vi "Offline Noise Reduction with Time Varying Filter.vi"() -> ()   [LabVIEW 2023]
doc: "This example shows the application of linear Time Frequency Analysis VIs in offline noise reduction applications. \n\nFor nonstationary signals whose spectral contents evolve over time, you usually use time-varying filters to reduce noise in the signals. The specification of a time-varying filter changes over time and is adaptable to signals. The Time Varying Filter (Thresholding) Express VI implements filtering with the following three steps: converting a signal into the time-frequency representation using the Gabor transform, removing noise in the time-frequency domain, and reconstructing the signal with noise reduced using the Gabor expansion. The Gabor transform-based filtering can be applied to both online and offline applications. \n\nThis example uses the Time Varying Filter (Thresholding) Express VI to reduce noise in a simulated chirp signal. \n\n<b>Instructions:</b>\n1) Run this VI.\n2) Compare the original <b>Noisy Signal</b> and <b>Denoised Signal</b>.\n3) Browse the Block Diagram of this example and double-click the Time Varying Filter (Thresholding) Express VI to observe the settings of the time-varying filter."
uses:
  <vilib>/addons/Time Frequency Analysis/typedefs.llb/TFA Data.ctl
  Instance           1 56Saved   Offline Noise Reduction with Time Varying Filter .vi
  <vilib>/addons/_Advanced Signal Processing/NI_AdvSigProcTFA.lvlib
panel:
  out "aspt-left-top":bool
  out "Signals":waveform(dbl)[](graph)
  # "Overview: Shows the application of linear Time Frequency Analysis VIs in offline noise reduction applications.\nRequirements: LabVIEW Full Development System, Advanced Signal Processing Toolkit\nInstructions: \n1. Run this VI.\n2. Compare the original Noisy Signal and Denoised Signal.\n3. Browse the block diagram of this example and double-click the Time Varying Filter (Thresholding) Express VI to observe the settings of the time-varying filter."
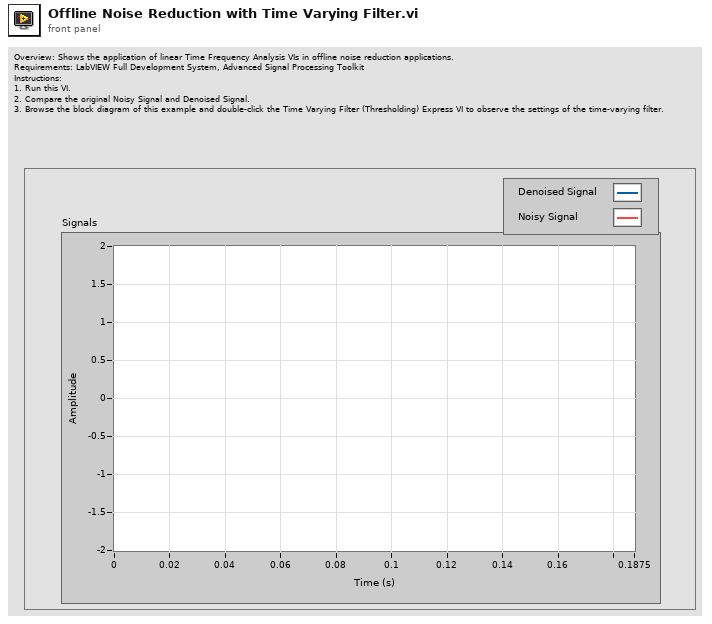
[diagram p1: front panel]
types:
  T1 = typedef "NI_AdvSigProcTFA.lvlib/TFA Data.ctl" = u16
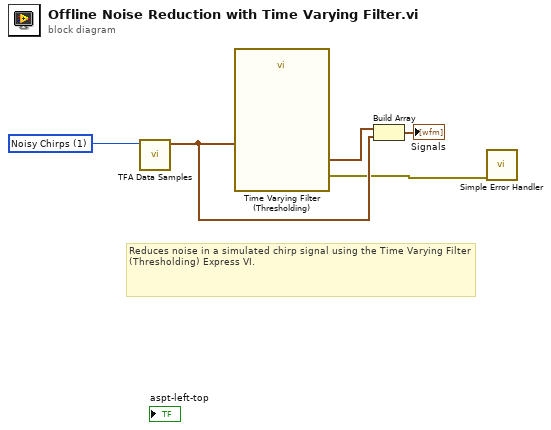
[diagram p0: block diagram]
diagram:
  w2 = T1 1 items=["PC Fan"=0, "Noisy Chirps"=1, "TDR 1"=2, "TDR 2"=3, "Liquefaction"=4, "Liquefaction Free"=5, "Aneurysm"=6, "Bat"=7, "RF"=8, "Two Gaussian"=9, "Three Gaussian"=10, "Chirp"=11, "Gaussian Chirp"=12, "Cross Chirp"=13, "Doppler"=14, "HOP"=15, "TF Sine"=16, "Three Tone"=17, "Four Tone"=23, "Blood Flow Doppler (phase a)"=20, "Blood Flow Doppler (phase b)"=21, "Heart sound"=22, "-"=18, "Random Noise"=19] ("data")
  # "Reduces noise in a simulated chirp signal using the Time Varying Filter (Thresholding) Express VI."
  n1 = call <vilib>:"TFA Data Samples.vi"("data"=w2) -> ("signal"=w5:waveform(dbl))  [unwired: 10 out]
  n2 = call "Time Varying Filter (Thresholding)"("Signal"=w5) -> ("error out"=w1:errorcluster, "Filtered Signal"=w4:waveform(dbl))  [unwired: 1 in, 8 out]
  n3 = Build Array(w4, w5) -> (→"Signals":waveform(dbl)[])
  n4 = call <vilib>:"Simple Error Handler.vi"("error in (no error)"=w1) -> ()  [unwired: 4 in, 5 out]
